vi "Describe Call Comparison.vi"(10 "VI Call 2":T1, 11 "VI Call 1":T1) -> (3 "delimited string":string)   [LabVIEW 2020, in "String Input Matching Comparator.lvclass"]
uses:
  String Input Matching Comparator.lvclass
  String Input Matching Comparator.lvclass/String Input Matching Comparator.ctl
  Core/Comparator/Comparator.lvclass
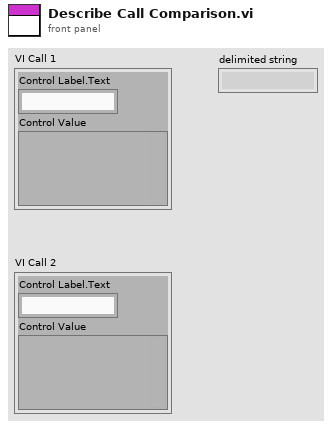
[diagram p1: front panel]
types:
  T1 = cluster{"Control Label.Text":string, "Control Value":variant}
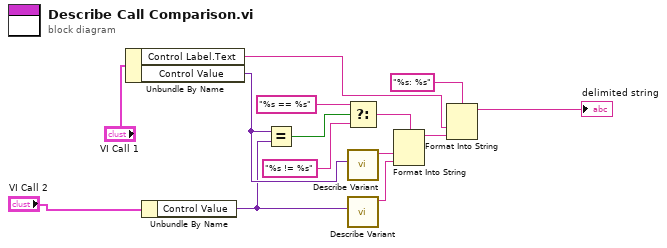
[diagram p0: block diagram]
diagram:
  n1 = Unbundle By Name("VI Call 1") -> ("Control Label.Text"=w8:string, "Control Value"=w13:variant)
  n2 = Unbundle By Name("VI Call 2") -> ("Control Value"=w12:variant)
  n3 = Equal?(x=w13, y=w12) -> (x = y?=w11:bool)
  n4 = Select(t="%s == %s", s=w11, f="%s != %s") -> (s? t:f=w5:string)
  n5 = call "Describe Variant.vi"("Variant"=w13) -> ("Description with Type"=w6:string)  [unwired: 8 in, 2 out]
  n6 = call "Describe Variant.vi"("Variant"=w12) -> ("Description with Type"=w7:string)  [unwired: 8 in, 2 out]
  n7 = Format Into String(format string=w5, w6, w7) -> (resulting string=w9:string)  [unwired: 2 in, 1 out]
  n8 = Format Into String(format string="%s: %s", w8, w9) -> (resulting string=→"delimited string":string)  [unwired: 2 in, 1 out]
